vi "Toolbar Set Button Complete.vi"(0 "Display State In":T3={"Buttons Displayed"=0, "Button States"=[], "Button Size"=0, "Button Style"=enum."Classic", "Active Button"=0, "Force Regen?"=FALSE, "Tip String Ref"=refnum}, 1 "Index":i32, 2 "Disabled Picture":picture, 5 "State":T2, 7 "Type":T1, 9 "Container State":T5, 11 "error in (no error)":errorcluster, 12 "Off Picture":picture, 13 "On Picture":picture, 14 "Hover Picture":picture) -> (4 "Display State Out":T3={"Buttons Displayed"=0, "Button States"=[], "Button Size"=0, "Button Style"=enum."Classic", "Active Button"=0, "Force Regen?"=FALSE, "Tip String Ref"=refnum}, 15 "error out":errorcluster)   [LabVIEW 2012, in "Toolbar.xctl"]
doc: "Set a toolbar button paraneters with indivudal controls for each parameter"
uses:
  Toolbar.xctl
  <vilib>/_xctls/Container State.ctl
  Toolbar State.ctl
  Button_Class/Button.lvclass
  Button_Class/Type Defs/Button Style.ctl
  Button_Class/Type Defs/Button Status.ctl
  Button_Class/Type Defs/Button Type.ctl
  <vilib>/_xctls/XControlSupport.lvlib
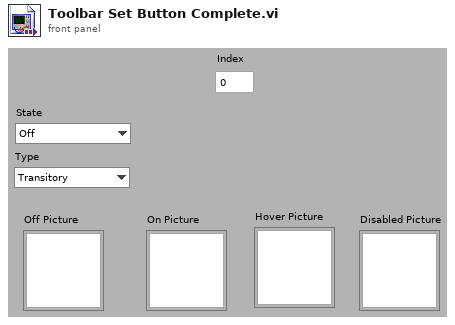
[diagram p1: front panel]
types:
  T1 = typedef "Button.lvclass/Button Type.ctl" = enum16{"Transitory", "Latching"}
  T2 = typedef "Button.lvclass/Button Status.ctl" = enum16{"Off", "Hover", "On", "Disabled"}
  T3 = typedef "Toolbar.xctl/Toolbar State.ctl" = cluster{"Buttons Displayed":i32, "Button States":refnum<class "Button.lvclass">[], "Button Size":i32, "Button Style":T4, "Active Button":i32, "Force Regen?":bool, "Tip String Ref":refnum<vi>}
  T4 = typedef "Button.lvclass/Button Style.ctl" = enum16{"System", "Modern", "Classic", "Rounded", "Silver", "Ni Theme", "Metallic"}
  T5 = typedef "XControlSupport.lvlib/Container State.ctl" = cluster{"Indicator?":bool, "Run Mode?":bool, " Refnum":refnum<vi>}
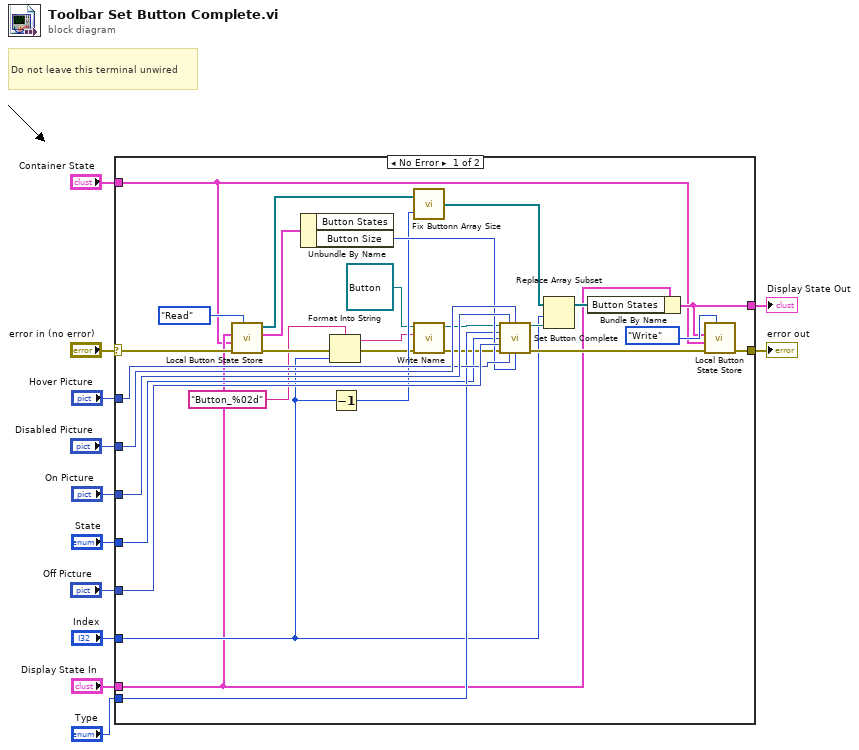
[diagram p0: block diagram]
diagram:
  # "Do not leave this terminal unwired"
  n1 = case shown="No Error" "error in (no error)" {
    selector: "error in (no error)" -> [w27 w43]
    tunnel: [w26 w43] -> w11
    tunnel: [w15 w42] -> w10
    tunnel: "Display State In" -> [w17 w42]
    tunnel: "Index" -> [w21 _]
    tunnel: "On Picture" -> [w40 _]
    tunnel: "Hover Picture" -> [w37 _]
    tunnel: "Type" -> [w35 _]
    tunnel: "State" -> [w34 _]
    tunnel: "Off Picture" -> [w39 _]
    tunnel: "Disabled Picture" -> [w38 _]
    tunnel: "Container State" -> [w14 _]
    frame No Error {
      n2 = call "Local Button State Store.vi"("Operation"=enum16{"Read", "Write"}."Read", "error in (no error)"=w27, "Container State"=w14, "Display State In"=w17) -> ("error out"=w23:errorcluster, "Display State Out"=w16:T3, "Button States"=w13:refnum<class "Button.lvclass">[])  [unwired: 5 out]
      n3 = Unbundle By Name(w16) -> ("Button Size"=w36:i32)  [unwired: 1 out]
      n4 = Format Into String(format string="Button_%02d", error in=w23, w21) -> (resulting string=w19:string, error out=w22:errorcluster)  [unwired: 1 in]
      n5 = Decrement(x=w21) -> (x-1=w32:i32)
      n6 = call "Fix Buttonn Array Size.vi"("Number of Buttons"=w32, "Button States In"=w13) -> ("Button States Out"=w33:refnum<class "Button.lvclass">[])
      n7 = call-dynamic "Write Name.vi"("error in (no error)"=w22, "Name"=w19, "Button.lvclass in"=refnum<class "Button.lvclass"> refnum) -> ("error out"=w25:errorcluster, "Button.lvclass out"=w24:refnum<class "Button.lvclass">)  [unwired: 7 out]
      n8 = call "Set Button Complete.vi"("Button in"=w24, "On Picture"=w40, "Disabled Picture"=w38, "Type"=w35, "State"=w34, "Off Picture"=w39, "error in (no error)"=w25, "Hover Picture"=w37, "Button Size"=w36) -> ("Button out"=w41:refnum<class "Button.lvclass">, "error out"=w28:errorcluster)  [unwired: 5 out]
      n9 = Replace Array Subset(array=w33, new element=w41, index=w21) -> (w30:refnum<class "Button.lvclass">[])
      n10 = Bundle By Name(cluster=w17, "Button States"=w30) -> (w15:T3)
      n11 = call "Local Button State Store.vi"("Operation"=enum16{"Read", "Write"}."Write", "error in (no error)"=w28, "Container State"=w14, "Display State In"=w15) -> ("error out"=w26:errorcluster)  [unwired: 1 in, 6 out]
    }
    frame Error {
    }
  }
  "Display State Out" <- w10
  "error out" <- w11
